vi "Find SLSC Module Custom Device by Name.vi"(8 "error in (no error)":errorcluster, 10 "Name":string, 11 "Target in":refnum<k24>) -> (0 "error out":errorcluster, 2 "CD Ref":T1 format="%.0x", 3 "Target out":refnum<k24>)   [LabVIEW 2017, in "SLSC Switch Scripting.lvlib"]
uses:
  SLSC Switch Scripting.lvlib
  NationalInstruments.VeriStand.SystemDefinitionAPI
  <vilib>/NI Veristand/Custom Device API/Custom Device Item Ref.ctl
  <vilib>/NI VeriStand/Custom Device API/Custom Device API.lvlib
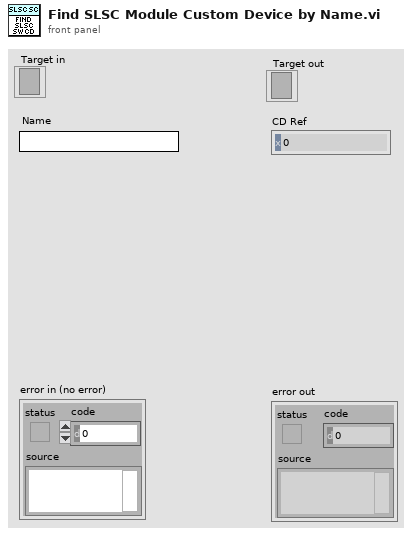
[diagram p1: front panel]
types:
  T1 = typedef "Custom Device API.lvlib/Custom Device Item Ref.ctl" = u64
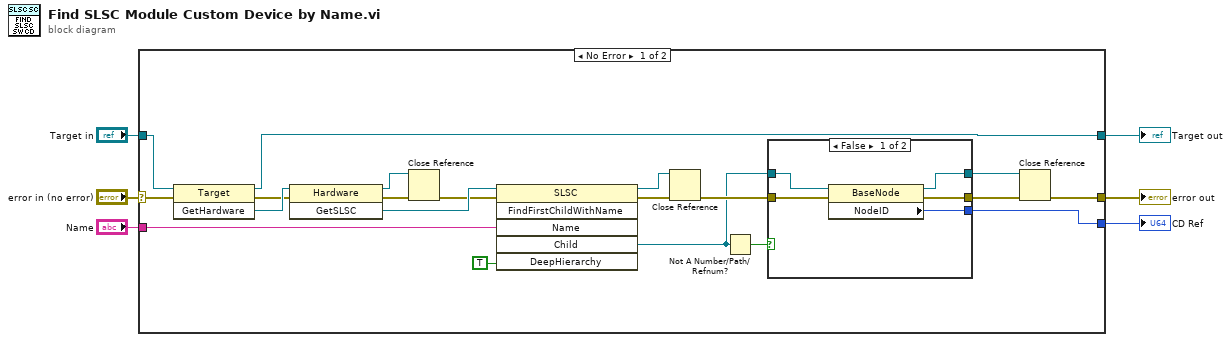
[diagram p0: block diagram]
diagram:
  n1 = case shown="No Error" "error in (no error)" {
    selector: "error in (no error)" -> [w26 w35]
    tunnel: [w14 w35] -> w6
    tunnel: "Target in" -> [w25 w34]
    tunnel: [w19 w34] -> w3
    tunnel: "Name" -> [w23 _]
    tunnel: [w16 _] -> w1
    frame No Error {
      n2 = invoke class="Target" method="GetHardware"(reference=w25, error in=w26) -> (reference out=w19:refnum<k24>, error out=w8:errorcluster, "GetHardware"=w12:refnum<k24>)  [unwired: 1 in]
      n3 = invoke class="Hardware" method="GetSLSC"(reference=w12, error in=w8) -> (reference out=w10:refnum<k24>, error out=w7:errorcluster, "GetSLSC"=w11:refnum<k24>)  [unwired: 1 in]
      n4 = Close Reference(reference=w10, error in (no error)=w7) -> (error out=w9:errorcluster)
      n5 = invoke class="SLSC" method="FindFirstChildWithName"(reference=w11, error in=w9, "Name"=w23, "DeepHierarchy"=TRUE) -> (reference out=w22:refnum<k24>, error out=w21:errorcluster, "Child"=w18:refnum<k24>)  [unwired: 2 in, 3 out]
      n6 = Close Reference(reference=w22, error in (no error)=w21) -> (error out=w20:errorcluster)
      n7 = Not A Number/Path/Refnum?(number/path/refnum=w18) -> (NaN/Path/Refnum?=w17:bool)
      n8 = case shown="False" w17 {
        tunnel: [w27 w33] -> w13
        tunnel: w20 -> [w29 w33]
        tunnel: w18 -> [w31 w32]
        tunnel: [w30 _] -> w16
        tunnel: [w28 w32] -> w15
        frame False {
          n9 = property class="BaseNode"(reference=w31, error in=w29) -> (reference out=w28:refnum<k24>, error out=w27:errorcluster, "NodeID"=w30:u64)
        }
        frame True {
        }
      }
      n10 = Close Reference(reference=w15, error in (no error)=w13) -> (error out=w14:errorcluster)
    }
    frame Error {
    }
  }
  "Target out" <- w3
  "error out" <- w6
  "CD Ref" <- w1
